vi "ws_templates export template.vi"(8 "error out":errorcluster, 10 "First Value":string, 11 "Connection Refnum":T1) -> (0 "error out 2":errorcluster, 1 "empty keyed array":T2, 2 "String":string, 3 "Connection Refnum 2":T1, 5 "Filename":string)   [LabVIEW 2011]
uses:
  SI.LIB/ODBC/SQL Controls/Connection Refnum.ctl
  <vilib>/addons/internet/utils/keyedarr.llb/Keyed Array.ctl
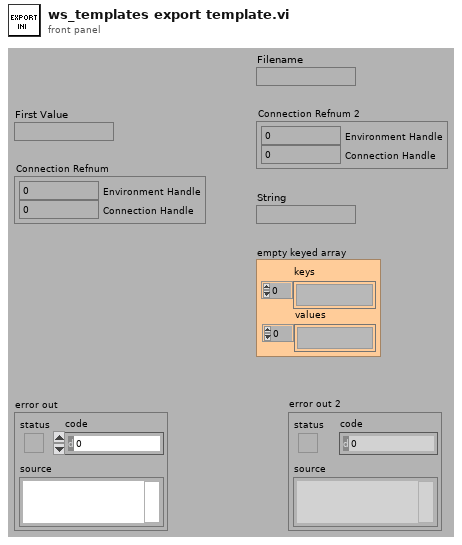
[diagram p1: front panel]
types:
  T1 = typedef "Connection Refnum.ctl" = cluster{"Environment Handle":i32, "Connection Handle":i32}
  T2 = typedef "Keyed Array.ctl" = cluster{"keys":string[], "values":string[]}
  T3 = enum16{"open", "replace", "create", "open or create", "replace or create", "replace or create with confirmation"}
  T4 = typedef "Template Record.ctl" = cluster{"ixTemplate":i32, "sxTemplateId":string, "sDescription":string, "sCreator":string, "tCreationDate":timestamp, "sModifier":string, "tModifiedDate":timestamp, "sType":string, "sStyle":string, "sFormat":string, "dWidth":dbl, "dHeight":dbl, "sFilename":string, "sScript":string, "sLayout":string, "sEditor":string, "sStyleProcess":string}
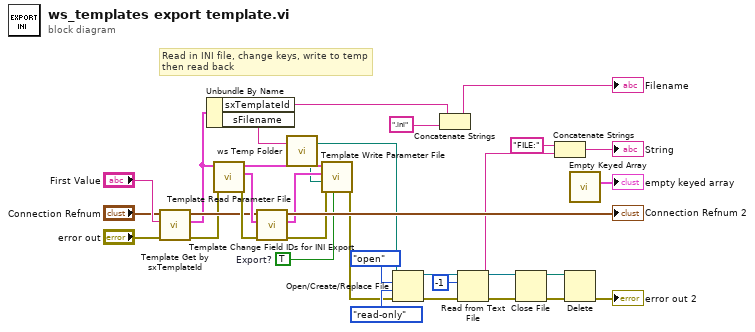
[diagram p0: block diagram]
diagram:
  w30 = TRUE  # Export?
  # "Read in INI file, change keys, write to temp\nthen read back"
  n1 = call "Template Get by sxTemplateId.vi"("error in (no error)"="error out", "sxTemplateId (\"\")"="First Value", "Connection Refnum"="Connection Refnum") -> ("error out"=w21:errorcluster, "Template Record"=w22:T4, "Connection Refnum"=w25:T1)  [unwired: 6 out]
  n2 = Unbundle By Name(w22) -> ("sxTemplateId"=w3:string, "sFilename"=w31:string)
  n3 = call "Template Read Parameter File.vi"("error in (no error)"=w21, "Template Record"=w22) -> ("error out"=w26:errorcluster, "Parameters"=w27:T2, "updated Template Record"=w33:T4)  [unwired: 1 in, 6 out]
  n4 = call "Template Change Field IDs for INI Export.vi"("error in (no error)"=w26, "Parameters"=w27, "Connection Refnum"=w25) -> ("error out"=w29:errorcluster, "Parameters 2"=w28:T2, "Connection Refnum 2"=→"Connection Refnum 2":T1)  [unwired: 6 out]
  n5 = call "ws Temp Folder.vi"("Relative Path (\"\")"=w31) -> ("Temp Folder"=w9:path)  [unwired: 2 in]
  n6 = call "Template Write Parameter File.vi"("Export?"=w30, "error in (no error)"=w29, "Export Path (\"\")"=w9, "Parameters (empty)"=w28, "Template Record"=w33) -> ("error out"=w8:errorcluster)  [unwired: 1 in, 5 out]
  n7 = Open/Create/Replace File(file path (use dialog)=w9, error in=w8, operation (0:open)=T3."open", access (0:read/write)=enum16{"read/write", "read-only", "write-only"}."read-only") -> (refnum out=w15:refnum<file>, error out=w10:errorcluster)  [unwired: 3 out]
  n8 = Concatenate Strings(w3, ".ini") -> (→"Filename":string)
  n9 = Read from Text File(file (use dialog)=w15, count=-1, error in=w10) -> (refnum out=w12:refnum<file>, text=w7:string, error out=w11:errorcluster)  [unwired: 2 out]
  n10 = Close File(refnum=w12, error in=w11) -> (path=w4:path, error out=w6:errorcluster)
  n11 = Concatenate Strings("FILE:", w7) -> (→"String":string)
  n12 = Delete(path (use dialog)=w4, error in=w6) -> (error out=→"error out 2":errorcluster)  [unwired: 5 out]
  n13 = call "Empty Keyed Array.vi"() -> ("empty keyed array"=→"empty keyed array":T2)  [unwired: 3 out]
